vi "Client Storage.vi"(3 "Relative Path (\"\" - Folder)":string) -> (1 "Client Storage Path":path)   [LabVIEW 2011]
uses:
  <vilib>/Utility/sysdir.llb/System Directory Type.ctl
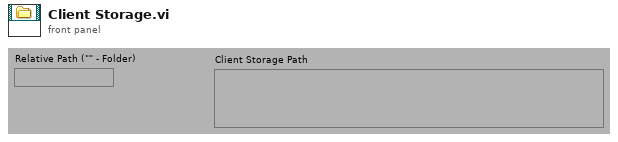
[diagram p1: front panel]
types:
  T1 = enum32{"invalid app kind", "Development System", "Run Time System", "Student Edition", "Embedded LabVIEW", "Evaluation", "Custom"}
  T2 = typedef "System Directory Type.ctl" = i32
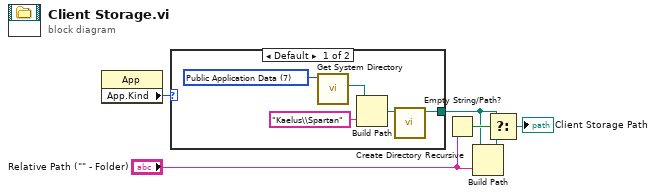
[diagram p0: block diagram]
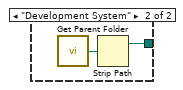
[diagram p2: hidden frame]
diagram:
  n1 = property class="App"() -> ("App.Kind"=w6:T1)  [unwired: 2 in, 2 out]
  n2 = case shown="Default" w6 {
    tunnel: [w7 w12] -> w2
    frame Default {
      w9 = T2 7 items=["User Home", "User Desktop", "User Documents", "User Application Data", "User Preferences", "User Temporary", "Public Documents", "Public Application Data", "Public Preferences", "System Core Libraries", "System Installed Libraries", "Application Files", "Boot Volume Root"] ("system directory type")
      n3 = call <vilib>:"Get System Directory.vi"("system directory type"=w9) -> ("system directory"=w8:path)  [unwired: 10 in]
      n4 = Build Path(base path=w8, name or relative path="Kaelus\\Spartan" ("time format string (%c)")) -> (appended path=w10:path)
      n5 = call <vilib>:"Create Directory Recursive.vi"("directory"=w10) -> ("directory copy"=w7:path)  [unwired: 2 in, 4 out]
    }
    frame "Development System" {
      n6 = call "Get Parent Folder.vi"() -> ("path"=w13:path)  [unwired: 5 out]
      n7 = Strip Path(path=w13) -> (stripped path=w12:path)  [unwired: 1 out]
    }
  }
  n8 = Empty String/Path?(string/path="Relative Path (\"\" - Folder)") -> (empty?=w5:bool)
  n9 = Build Path(base path=w2, name or relative path="Relative Path (\"\" - Folder)") -> (appended path=w4:path)
  n10 = Select(t=w2, s=w5, f=w4) -> (s? t:f=→"Client Storage Path":path)
